vi "log.vi"(9 "Car Wash Type":string, 10 "remote port or service name":u16, 11 "timeout ms (60000)":i32) -> ()   [LabVIEW 2024]
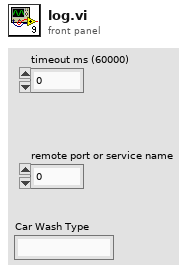
[diagram p1: front panel]
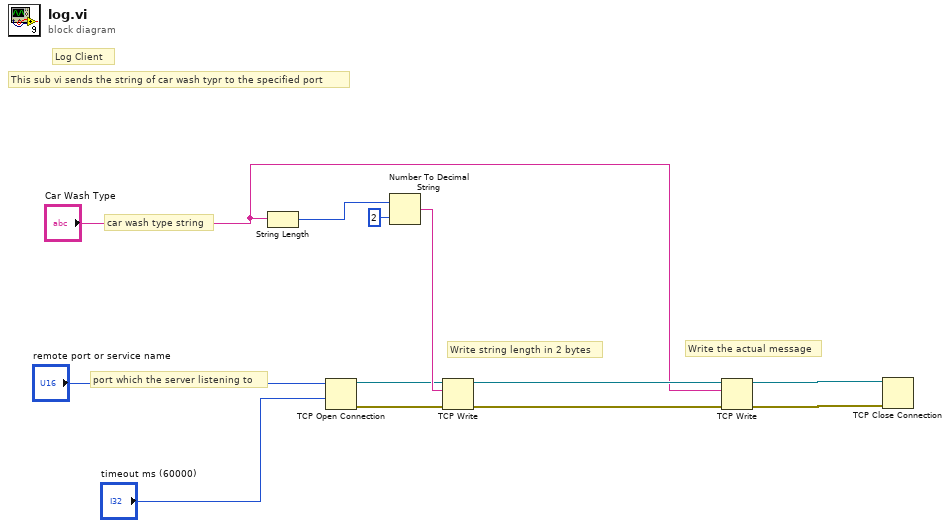
[diagram p0: block diagram]
diagram:
  # "Write the actual message"
  # "Write string length in 2 bytes"
  # "This sub vi sends the string of car wash typr to the specified port"
  # "Log Client"
  # "port which the server listening to"
  # "car wash type string"
  n1 = String Length(string="Car Wash Type") -> (length=w9:i32)
  n2 = TCP Open Connection(remote port or service name="remote port or service name", timeout ms (60000)="timeout ms (60000)") -> (connection ID=w4:refnum<k5>, error out=w6:errorcluster)  [unwired: 3 in]
  n3 = Number To Decimal String(number=w9, width (-)=i16 2) -> (decimal integer string=w10:string)
  n4 = TCP Write(connection ID=w4, data in=w10, error in (no error)=w6) -> (connection ID out=w5:refnum<k5>, error out=w7:errorcluster)  [unwired: 1 in, 1 out]
  n5 = TCP Write(connection ID=w5, data in="Car Wash Type", error in (no error)=w7) -> (connection ID out=w11:refnum<k5>, error out=w12:errorcluster)  [unwired: 1 in, 1 out]
  n6 = TCP Close Connection(connection ID=w11, error in (no error)=w12) -> ()  [unwired: 1 in, 2 out]
